vi "dvp Vi Get Noise Reduct2d.vi"(10 "pNoiseReduct2d":i32, 11 "handle":u32) -> (2 "pNoiseReduct2d out":i32, 3 "function return":u32(ring))   [LabVIEW 2018, in "LabViewDVPCamera.lvlib"]
doc: "LabviewDvp2Api dvpStatus dvpViGetNoiseReduct2d(dvpHandle handle, dvpInt32 *pNoiseReduct2d);"
uses:
  LabViewDVPCamera.lvlib
  LabViewDVPCamera/LabViewDVPCamera.dll
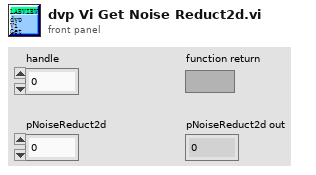
[diagram p1: front panel]
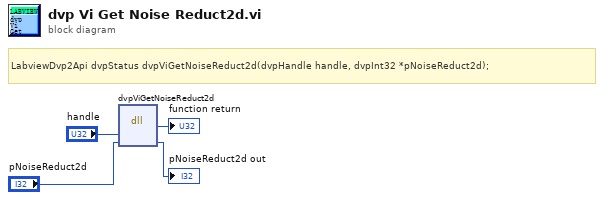
[diagram p0: block diagram]
diagram:
  # "LabviewDvp2Api dvpStatus dvpViGetNoiseReduct2d(dvpHandle handle, dvpInt32 *pNoiseReduct2d);"
  n1 = dll-call lib="C:/Program Files (x86)/DVP2 Labview cn 64/Sample/LabViewDVPCamera/LabViewDVPCamera.*" fn="dvpViGetNoiseReduct2d"("handle"="handle", "pNoiseReduct2d"="pNoiseReduct2d") -> (→"function return":u32, "pNoiseReduct2d"=→"pNoiseReduct2d out":i32)  [unwired: 4 in, 2 out]
